vi "AdjustLeftRightSpeeds.vi"() -> ()   [LabVIEW 2017]
panel:
  out "Right":dbl
  out "Left":dbl
  in  "Trackwidth":dbl
  in  "Right":dbl
  in  "Left":dbl
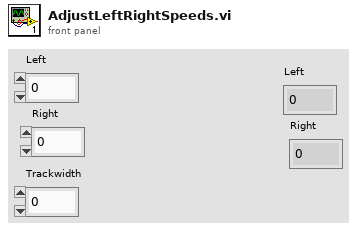
[diagram p1: front panel]
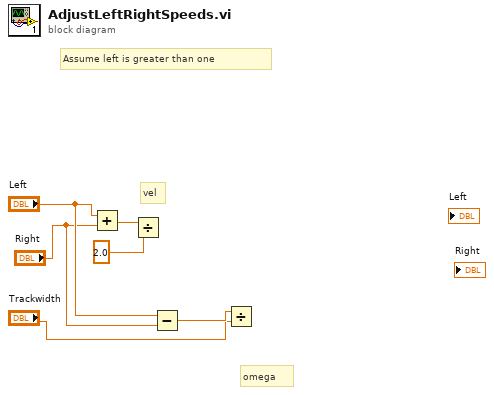
[diagram p0: block diagram]
diagram:
  # "omega"
  # "vel"
  # "Assume left is greater than one"
  n1 = Add(x="Left", y="Right") -> (x+y=w6:dbl)
  n2 = Divide(x=w6, y=2.0) -> ()  [unwired: 1 out]
  n3 = Subtract(x="Left", y="Right") -> (x-y=w2:dbl)
  n4 = Divide(x=w2, y="Trackwidth") -> ()  [unwired: 1 out]
